vi "Construct URI.vi"(6 "Arguments":cluster{"key":string, "value":string}[](array[cluster]), 8 "path":string, 9 "port":string, 10 "address":string, 11 "protocol":string) -> (3 "URI":string="opc.tcp://localhost:49580")   [LabVIEW 2021, in "smo.lvlib" / "URI.lvlib"]
uses:
  URI.lvlib
  <vilib>/regexp/Match Regular Expression.xnode
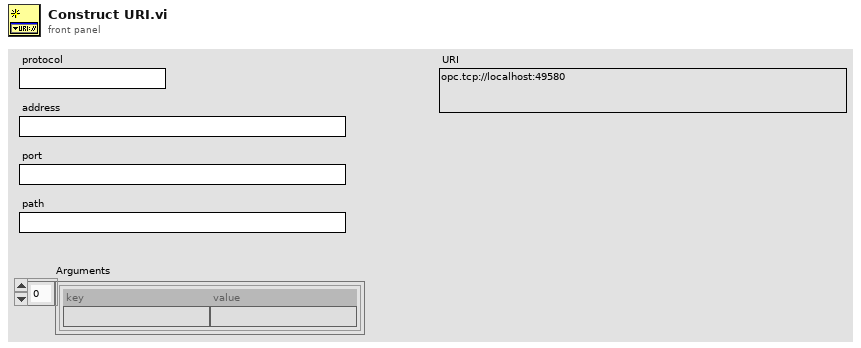
[diagram p1: front panel]
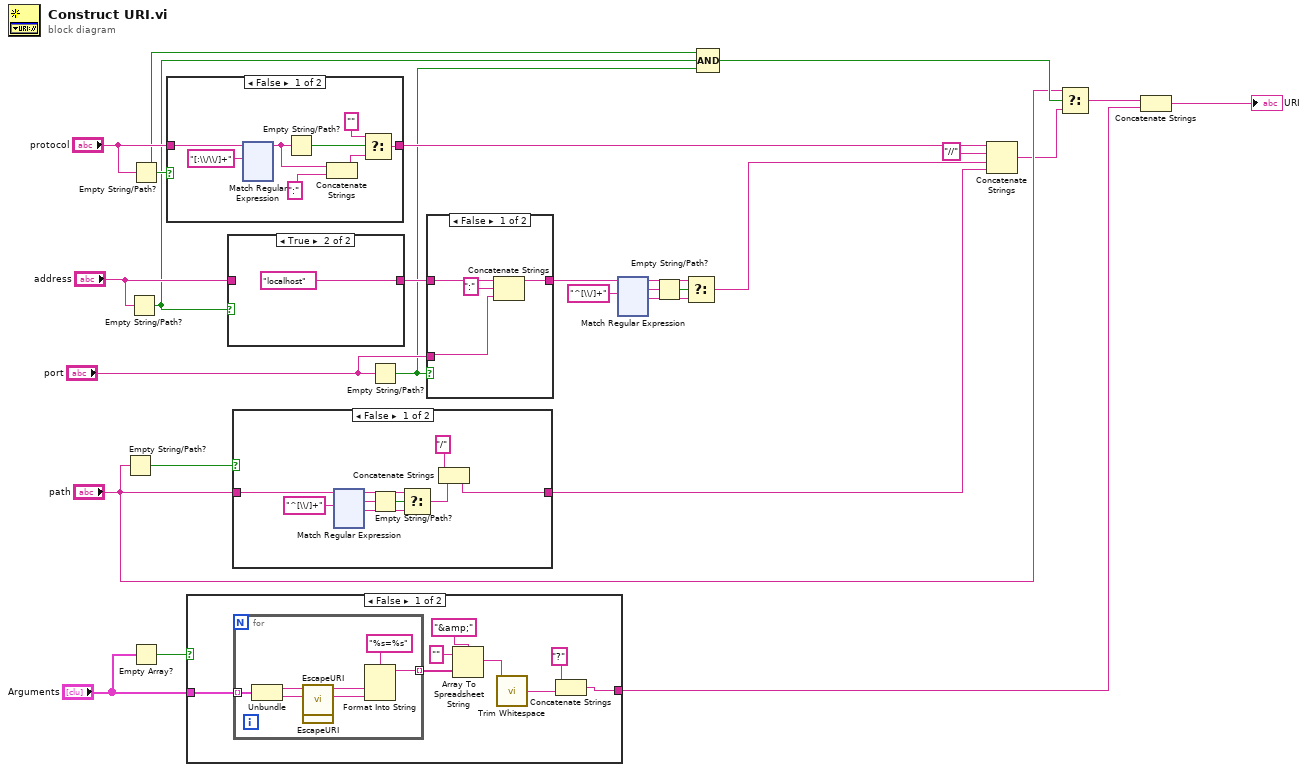
[diagram p0: block diagram]
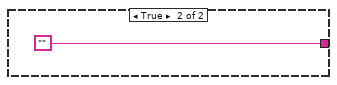
[diagram p2: hidden frame]
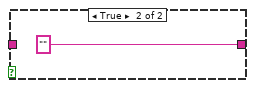
[diagram p6: hidden frame]
diagram:
  n1 = Empty String/Path?(string/path="path") -> (empty?=w3:bool)
  n2 = Empty String/Path?(string/path="address") -> (empty?=w4:bool)
  n3 = Empty String/Path?(string/path="protocol") -> (empty?=w21:bool)
  n4 = Empty Array?(array="Arguments") -> (empty?=w8:bool)
  n5 = case shown="False" w21 {
    tunnel: "protocol" -> [w33 _]
    tunnel: [w30 "" ("t")] -> w25
    frame False {
      n6 = xnode "Match Regular Expression"("input string"=w33, "regular expression"="[:\\/\\/]+") -> ("before match"=w28:string)  [unwired: 4 in, 4 out]
      n7 = Empty String/Path?(string/path=w28) -> (empty?=w32:bool)
      n8 = Concatenate Strings(w28, ":" ("t")) -> (w29:string)
      n9 = Select(t="", s=w32, f=w29) -> (s? t:f=w30:string)
    }
    frame True {
    }
  }
  n10 = case shown="False" w8 {
    tunnel: "Arguments" -> [w160 _]
    tunnel: [w153 ""] -> w7
    frame False {
      n11 = for {
        tunnel: w160 -> [w167] mode=indexing
        tunnel: [w165] -> w159 mode=indexing
        n12 = Unbundle(w167) -> ("key"=w164:string, "value"=w163:string)
        n13 = call "EscapeURI.vi"("URI"=w164) -> ("Escaped URI"=w161:string)  [unwired: 10 in]
        n14 = call "EscapeURI.vi"("URI"=w163) -> ("Escaped URI"=w162:string)  [unwired: 10 in]
        n15 = Format Into String(format string="%s=%s", w161, w162) -> (resulting string=w165:string)  [unwired: 2 in, 1 out]
      }
      n16 = Array To Spreadsheet String(delimiter (Tab)="&amp;", array=w159, 3:"" ("format string")) -> (spreadsheet string=w156:string)
      n17 = call <vilib>:"Trim Whitespace.vi"("string"=w156) -> ("trimmed string"=w154:string)  [unwired: 1 in]
      n18 = Concatenate Strings("?" ("t"), w154) -> (w153:string)
    }
    frame True {
    }
  }
  n19 = case shown="True" w4 {
    tunnel: [w169 "localhost" ("t")] -> w23
    tunnel: "address" -> [w169 _]
    frame False {
    }
    frame True {
    }
  }
  n20 = case shown="False" w3 {
    tunnel: "path" -> [w172 w297]
    tunnel: [w178 w297] -> w22
    frame False {
      n21 = xnode "Match Regular Expression"("input string"=w172, "regular expression"="^[\\/]+") -> ("before match"=w175:string, "whole match"=w174:string, "after match"=w177:string)  [unwired: 4 in, 2 out]
      n22 = Empty String/Path?(string/path=w174) -> (empty?=w176:bool)
      n23 = Select(t=w175, s=w176, f=w177) -> (s? t:f=w171:string)
      n24 = Concatenate Strings("/" ("t"), w171) -> (w178:string)
    }
    frame True {
    }
  }
  n25 = Empty String/Path?(string/path="port") -> (empty?=w20:bool)
  n26 = case shown="False" w20 {
    tunnel: "port" -> [w298 _]
    tunnel: w23 -> [w301 w302]
    tunnel: [w300 w302] -> w12
    frame False {
      n27 = Concatenate Strings(w301, ":" ("t"), w298) -> (w300:string)
    }
    frame True {
    }
  }
  n28 = xnode "Match Regular Expression"("input string"=w12, "regular expression"="^[\\/]+") -> ("before match"=w14:string, "whole match"=w15:string, "after match"=w11:string)  [unwired: 4 in, 2 out]
  n29 = Empty String/Path?(string/path=w15) -> (empty?=w13:bool)
  n30 = Select(t=w14, s=w13, f=w11) -> (s? t:f=w1:string)
  n31 = Compound Arithmetic op=AND(w21, w4, w20) -> (w19:bool)
  n32 = Concatenate Strings(w25, "//" ("t"), w1, w22) -> (w17:string)
  n33 = Select(t="path", s=w19, f=w17) -> (s? t:f=w6:string)
  n34 = Concatenate Strings(w6, w7) -> (→"URI":string)
